vi "例4-10.vi"() -> ()   [LabVIEW 2019]
panel:
  out "组合字符串长度":dbl
  out "组合字符串":string
  in  "单位":string="V"
  in  "数值":dbl=12.3
  in  "题头":string="Voltage="
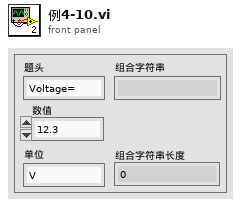
[diagram p1: front panel]
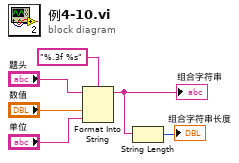
[diagram p0: block diagram]
diagram:
  n1 = Format Into String(format string="%.3f %s" ("格式字符串"), initial string="题头", "数值", "单位") -> (resulting string=w2:string)  [unwired: 1 in, 1 out]
  "组合字符串" <- w2
  n2 = String Length(string=w2) -> (length=→"组合字符串长度":i32)
